vi "Publish N Per-Site Data.vi"(7 "Published Data Id":tag[](array[tag]), 8 "error in (no error)":errorcluster, 9 "Data In":dbl[][](array[numeric]), 10 "Pin":tag, 11 "Semiconductor Module Context":T1) -> (0 "error out":errorcluster, 3 "Semiconductor Module Context Out":T1)   [LabVIEW 2020]
uses:
  <vilib>/NI_TestStand_SemiconductorModule/NI_TestStand_Semiconductor_Module.lvlibp/PinMap/General/SemiconductorModuleContext.ctl
  <vilib>/NI_TestStand_SemiconductorModule/NI_TestStand_Semiconductor_Module.lvlibp/PinMap/General/Publish/PublishDataDoubleFunctionalTest.vi
  <vilib>/NI_TestStand_SemiconductorModule/NI_TestStand_Semiconductor_Module.lvlibp
panel:
  # "Rows - per Publish Id\nCols - Site data"
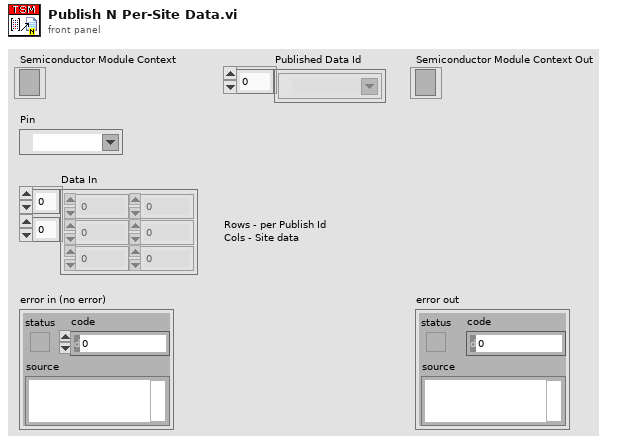
[diagram p1: front panel]
types:
  T1 = typedef "NI_TestStand_Semiconductor_Module.lvlibp/SemiconductorModuleContext.ctl" = refnum<k7>
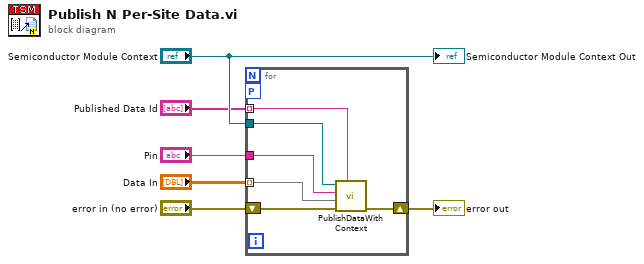
[diagram p0: block diagram]
diagram:
  n1 = for {
    tunnel: "Data In" -> [w11] mode=indexing
    shift-right: [w9] -> w4
    shift-left: "error in (no error)" -> [w12]
    workers-P: _ -> [_]
    tunnel: "Semiconductor Module Context" -> [w10]
    tunnel: "Pin" -> [w8]
    tunnel: "Published Data Id" -> [w7] mode=indexing
    n2 = call-poly <vilib>:"PublishDataWithContext.vi"("Published Data Id"=w7, "error in (no error)"=w12, "Data In"=w11, "Pin"=w8, "Semiconductor Module Context"=w10) -> ("error out"=w9:errorcluster)  [unwired: 5 in, 1 out]
  }
  "error out" <- w4
  "Semiconductor Module Context Out" <- "Semiconductor Module Context"
